vi "Format Main Status.vi"() -> (2 "FullStat":string, 3 "ShortStat":string)   [LabVIEW 2019]
uses:
  RT Controls/Top Dome Status.ctl
  RT Controls/Main Box Status.ctl
  RT Controls/Rotation Status.ctl
  RT Controls/Last Rotation.ctl
  RT Controls/Homing State.ctl
  RT Controls/Main Box Control.ctl
  RT Controls/Top Dome Control.ctl
  RT Controls/Main Box Config.ctl
  RT Controls/TopBox Config.ctl
  RT Controls/FPGA State.ctl
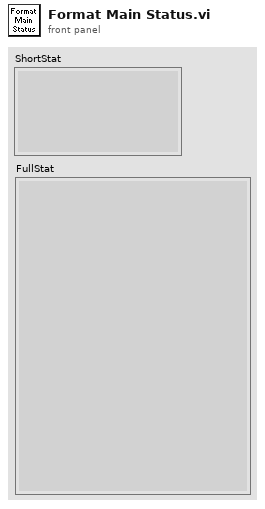
[diagram p1: front panel]
types:
  T1 = typedef "Main Box Config.ctl" = cluster{"WatchdogTim":i32, "DirRevDel":i32, "Coast":dbl, "HSThres":dbl, "EncCounts360":u64, "HomePos":dbl, "EncRefDeg":dbl, "EncRefCounts":u64, "Tol":dbl, "CloudEn":bool, "AutoShutEn":bool, "RainTim":i32, "AZTimeout":i32, "AZEncPol":enum16{"Positive", "Negative"}}
  T2 = typedef "Main Box Status.ctl" = cluster{"RotStatus":T3, "EMButton":bool, "TopComms":bool, "CurAZ":dbl, "At Home":bool, "LastRot":T4, "Cloud":bool, "CurAZEnc":u64, "LastAZ":dbl, "AutoShut":bool, "WDTime":bool, "HomeState":T5}
  T3 = typedef "Rotation Status.ctl" = enum16{"Stop", "Left", "Right", "Homing"}
  T4 = typedef "Last Rotation.ctl" = enum16{"--", "RR", "RL"}
  T5 = typedef "Homing State.ctl" = enum16{"Idle", "SlewFwd", "SlewRev", "SeekFwd", "SeekRev", "AtHome", "FwdWait", "RevWait"}
  T6 = typedef "Top Dome Status.ctl" = cluster{"UpperDoorStatus":enum16{"Ajar", "Open", "Shut", "Error"}, "LowerDoorStatus":enum16{"Ajar", "Shut", "Open", "Error"}, "EM Button":bool, "WDTime":bool, "AutoShut":bool, "Rain":bool, "Interlock":bool, "UpperDoorEl":dbl, "LowerDoorEl":dbl, "UpperDoorEnc":u64, "LowerDoorEnc":u64}
  T7 = typedef "Top Dome Control.ctl" = cluster{"OpenLowerDoor":bool, "CloseLowerDoor":bool, "OpenMainDoor":bool, "CloseMainDoor":bool}
  T8 = typedef "Main Box Control.ctl" = cluster{"ForwardDome":bool, "ReverseDome":bool, "GotoHome":bool, "HighSpeed":bool}
  T9 = typedef "FPGA State.ctl" = cluster{"mode request":enum16{"stop", "home", "position", "center"}, "az last rotation":enum16{"none", "forward", "reverse"}, "emergency stop":bool, "error?":bool, "errors":cluster{"emergency stop":bool, "encoder":bool, "az timeout":bool, "m1":bool, "m2":bool, "m4":bool}, "az enc counts":u64, "az pos":fxp<+/-,32,2>, "mode":u8, "sub mode":u8, "enc status":u16, "buttons":cluster{"em-stop":bool, "forward":bool, "reverse":bool, "open":bool, "close":bool, "up":bool, "down":bool, "force stop":bool}, "cloud?":bool, "cloud to counter":u32, "az to counter":u32, "env sensor":bool, "home sensor":bool, "rev dly counter":u32, "cmd request":i8, "cmd":i8, "config":cluster{"io.cloud-enable":bool, "io.encoder-negate":bool, "io.encoder-ref":u64, "io.encoder-step":u64, "io.home-pos":fxp<+/-,32,2>, "sm.az-timeout (ms)":u32, "sm.encoder-no-error":u16, "sm.main-pos-hs-thres":fxp<+/-,32,2>, "sm.main-pos-tol":fxp<+/-,32,2>, "sm.cloud-timeout (ms)":u32, "sm.rev-dly (ms)":u32, "io.encoder-center":u64, "sm-main-center-hs-thres":u64, "sm-main-center-tol":u64}, "homing?":bool, "homed?":bool, "az pos req":fxp<+/-,32,2>, "homing wait counter":u32, "config out":cluster{"io.cloud-enable":bool, "io.encoder-negate":bool, "io.encoder-ref":u64, "io.encoder-step":u64, "io.home-pos":fxp<+/-,32,2>, "sm.az-timeout (ms)":u32, "sm.encoder-no-error":u16, "sm.main-pos-hs-thres":fxp<+/-,32,2>, "sm.main-pos-tol":fxp<+/-,32,2>, "sm.cloud-timeout (ms)":u32, "sm.rev-dly (ms)":u32, "io.encoder-center":u64, "sm-main-center-hs-thres":u64, "sm-main-center-tol":u64}, "Chassis Temperature":i16}
  T10 = typedef "TopBox Config.ctl" = cluster{"WatchdogTim":i32, "RainEn":bool, "DoorMoveTO":i32, "AutoShutEn":bool, "DirRevDel":i32, "UpperClosedEnc":u64, "UpperOpenEnc":u64, "LowerClosedEnc":u64, "LowerOpenEnc":u64, "RainTim":i32, "DropoutTim":i32}
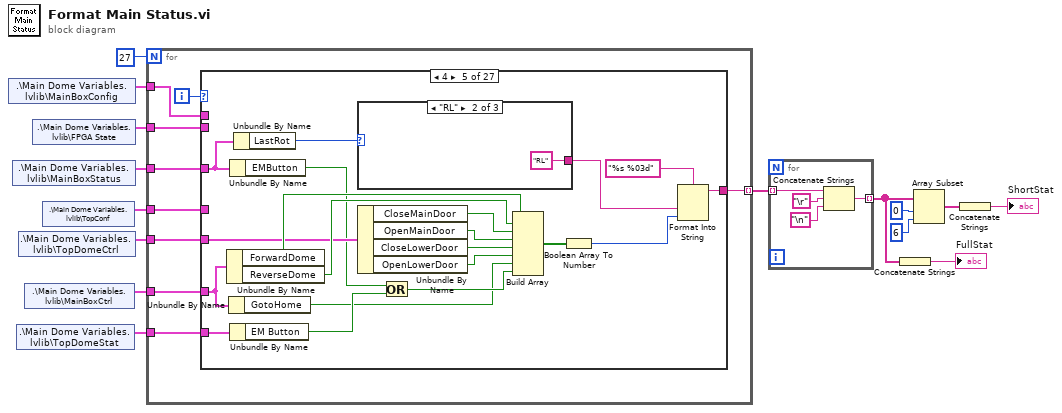
[diagram p0: block diagram]
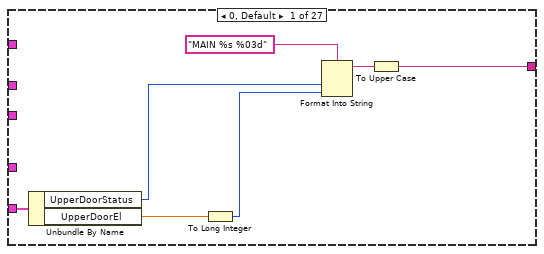
[diagram p2: hidden frame]
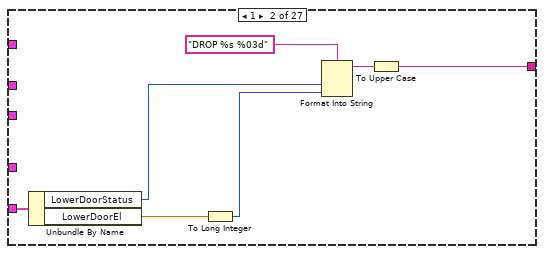
[diagram p3: hidden frame]
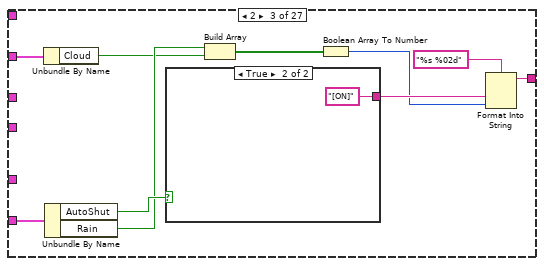
[diagram p4: hidden frame]
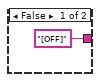
[diagram p5: hidden frame]
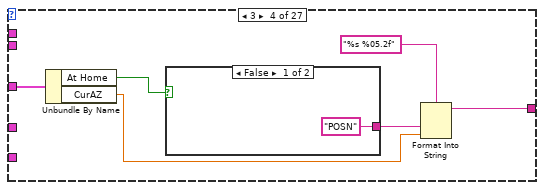
[diagram p6: hidden frame]
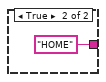
[diagram p7: hidden frame]
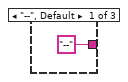
[diagram p8: hidden frame]
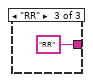
[diagram p9: hidden frame]
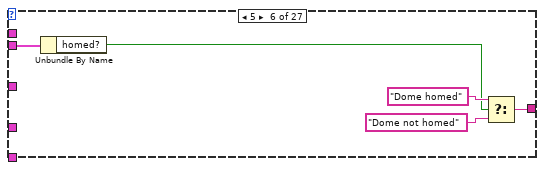
[diagram p10: hidden frame]
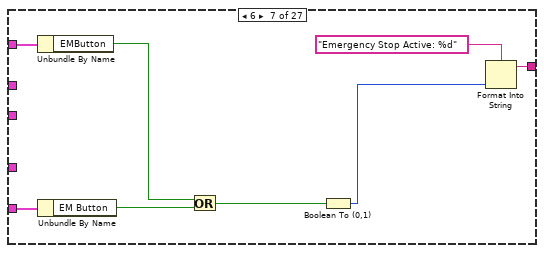
[diagram p11: hidden frame]
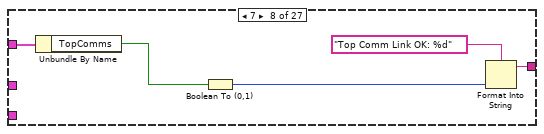
[diagram p12: hidden frame]
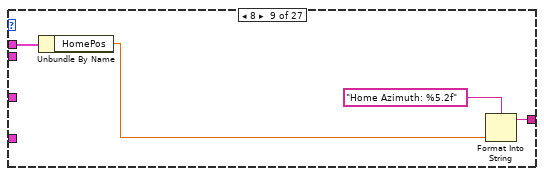
[diagram p13: hidden frame]
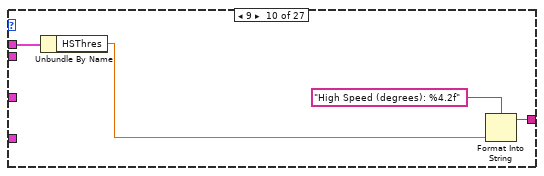
[diagram p14: hidden frame]
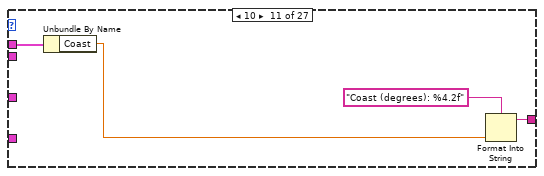
[diagram p15: hidden frame]
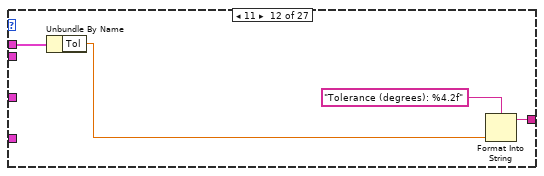
[diagram p16: hidden frame]
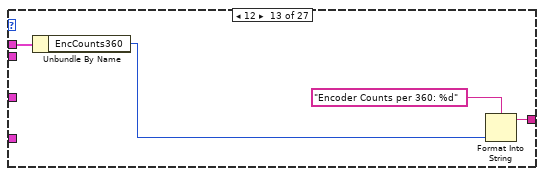
[diagram p17: hidden frame]
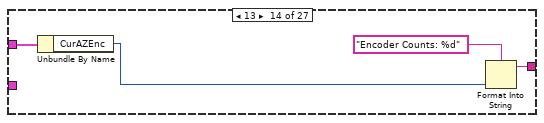
[diagram p18: hidden frame]
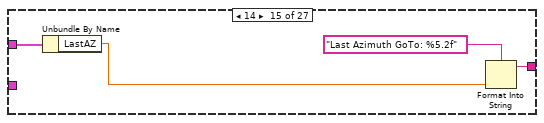
[diagram p19: hidden frame]
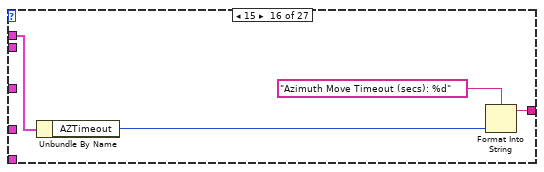
[diagram p20: hidden frame]
diagram:
  n1 = shared-variable ".\\Main Dome Variables.lvlib\\MainBoxConfig"() -> (w11:T1)  [unwired: 1 in, 1 out]
  n2 = shared-variable ".\\Main Dome Variables.lvlib\\MainBoxStatus"() -> (w14:T2)  [unwired: 1 in, 1 out]
  n3 = shared-variable ".\\Main Dome Variables.lvlib\\TopDomeStat"() -> (w15:T6)  [unwired: 1 in, 1 out]
  n4 = shared-variable ".\\Main Dome Variables.lvlib\\TopDomeCtrl"() -> (w12:T7)  [unwired: 1 in, 1 out]
  n5 = shared-variable ".\\Main Dome Variables.lvlib\\MainBoxCtrl"() -> (w13:T8)  [unwired: 1 in, 1 out]
  n6 = shared-variable ".\\Main Dome Variables.lvlib\\FPGA State"() -> (w1:T9)  [unwired: 1 in, 1 out]
  n7 = shared-variable ".\\Main Dome Variables.lvlib\\TopConf"() -> (w10:T10)  [unwired: 1 in, 1 out]
  n8 = for {
    N: 27 -> [_]
    tunnel: w15 -> [w24]
    tunnel: [w22] -> w5 mode=indexing
    tunnel: w14 -> [w21]
    tunnel: w13 -> [w20]
    tunnel: w12 -> [w19]
    tunnel: w11 -> [w18]
    tunnel: w10 -> [w17]
    tunnel: w1 -> [w16]
    i -> [w23]
    n9 = case shown="4" w23 {
      tunnel: w24 -> [w31 w38 w48 _ w67 _ w91 _ _ _ _ _ _ _ _ _ w134 _ _ _ _ _ _ _ _ _ _]
      tunnel: [w28 w35 w43 w51 w64 w85 w93 w98 w102 w106 w110 w114 w118 w122 w126 w130 w135 w140 w144 w148 w152 w156 w160 w164 w168 w172 w175] -> w22
      tunnel: w21 -> [_ _ w45 w56 w62 _ w92 w97 _ _ _ _ _ w120 w124 _ _ _ _ _ _ _ _ _ _ _ _]
      tunnel: w20 -> [_ _ _ _ w60 _ _ _ _ _ _ _ _ _ _ _ _ _ _ _ _ _ _ _ _ _ _]
      tunnel: w19 -> [_ _ _ _ w69 _ _ _ _ _ _ _ _ _ _ _ _ _ _ _ _ _ _ _ _ _ _]
      tunnel: w18 -> [_ _ _ _ _ _ _ _ w101 w105 w109 w113 w117 _ _ w128 _ w137 _ _ _ _ _ _ _ _ _]
      tunnel: w17 -> [_ _ _ _ _ _ _ _ _ _ _ _ _ _ _ _ _ _ w143 w147 w151 w155 w159 w163 w167 w171 _]
      tunnel: w16 -> [_ _ _ _ _ w83 _ _ _ _ _ _ _ _ _ _ _ _ _ _ _ _ _ _ _ _ w174]
      frame 0, Default {
        n10 = Unbundle By Name(w31) -> ("UpperDoorStatus"=w27:enum16{"Ajar", "Open", "Shut", "Error"}, "UpperDoorEl"=w26:dbl)
        n11 = To Long Integer(number=w26) -> (32bit integer=w25:i32)
        n12 = Format Into String(format string="MAIN %s %03d", w27, w25) -> (resulting string=w29:string)  [unwired: 2 in, 1 out]
        n13 = To Upper Case(1:w29) -> (0:w28:string)
      }
      frame 1 {
        n14 = Unbundle By Name(w38) -> ("LowerDoorStatus"=w34:enum16{"Ajar", "Shut", "Open", "Error"}, "LowerDoorEl"=w33:dbl)
        n15 = To Long Integer(number=w33) -> (32bit integer=w32:i32)
        n16 = Format Into String(format string="DROP %s %03d", w34, w32) -> (resulting string=w36:string)  [unwired: 2 in, 1 out]
        n17 = To Upper Case(1:w36) -> (0:w35:string)
      }
      frame 2 {
        n18 = Unbundle By Name(w45) -> ("Cloud"=w40:bool)
        n19 = Unbundle By Name(w48) -> ("AutoShut"=w47:bool, "Rain"=w41:bool)
        n20 = case shown="True" w47 {
          tunnel: ["[OFF]" ("string") "[ON]" ("string")] -> w44
          frame False {
          }
          frame True {
          }
        }
        n21 = Build Array(w41, w40) -> (w42:bool[])
        n22 = Boolean Array To Number(Boolean array=w42) -> (number=w39:u32)
        n23 = Format Into String(format string="%s %02d", w44, w39) -> (resulting string=w43:string)  [unwired: 2 in, 1 out]
      }
      frame 3 {
        n24 = Unbundle By Name(w56) -> ("At Home"=w55:bool, "CurAZ"=w52:dbl)
        n25 = case shown="False" w55 {
          tunnel: ["POSN" ("string") "HOME" ("string")] -> w54
          frame False {
          }
          frame True {
          }
        }
        n26 = Format Into String(format string="%s %05.2f", w54, w52) -> (resulting string=w51:string)  [unwired: 2 in, 1 out]
      }
      frame 4 {
        n27 = Unbundle By Name(w60) -> ("ForwardDome"=w75:bool, "ReverseDome"=w74:bool)
        n28 = Unbundle By Name(w60) -> ("GotoHome"=w59:bool)
        n29 = Unbundle By Name(w62) -> ("EMButton"=w61:bool)
        n30 = Unbundle By Name(w67) -> ("EM Button"=w63:bool)
        n31 = Unbundle By Name(w62) -> ("LastRot"=w78:T4)
        n32 = case shown="\"RL\"" w78 {
          tunnel: ["--" ("string") "RL" ("string") "RR" ("string")] -> w76
          frame "--", Default {
          }
          frame "RL" {
          }
          frame "RR" {
          }
        }
        n33 = Unbundle By Name(w69) -> ("CloseMainDoor"=w73:bool, "OpenMainDoor"=w72:bool, "CloseLowerDoor"=w71:bool, "OpenLowerDoor"=w70:bool)
        n34 = Or(x=w61, y=w63) -> (x .or. y?=w68:bool)
        n35 = Build Array(w75, w74, w73, w72, w71, w70, w59, w68) -> (w66:bool[])
        n36 = Boolean Array To Number(Boolean array=w66) -> (number=w65:u32)
        n37 = Format Into String(format string="%s %03d", w76, w65) -> (resulting string=w64:string)  [unwired: 2 in, 1 out]
      }
      frame 5 {
        n38 = Unbundle By Name(w83) -> ("homed?"=w82:bool)
        n39 = Select(t="Dome homed", s=w82, f="Dome not homed") -> (s? t:f=w85:string)
      }
      frame 6 {
        n40 = Unbundle By Name(w92) -> ("EMButton"=w88:bool)
        n41 = Unbundle By Name(w91) -> ("EM Button"=w87:bool)
        n42 = Or(x=w88, y=w87) -> (x .or. y?=w90:bool)
        n43 = Boolean To (0,1)(Boolean=w90) -> (0, 1=w89:i16)
        n44 = Format Into String(format string="Emergency Stop Active: %d", w89) -> (resulting string=w93:string)  [unwired: 2 in, 1 out]
      }
      frame 7 {
        n45 = Unbundle By Name(w97) -> ("TopComms"=w95:bool)
        n46 = Boolean To (0,1)(Boolean=w95) -> (0, 1=w96:i16)
        n47 = Format Into String(format string="Top Comm Link OK: %d", w96) -> (resulting string=w98:string)  [unwired: 2 in, 1 out]
      }
      frame 8 {
        n48 = Unbundle By Name(w101) -> ("HomePos"=w100:dbl)
        n49 = Format Into String(format string="Home Azimuth: %5.2f", w100) -> (resulting string=w102:string)  [unwired: 2 in, 1 out]
      }
      frame 9 {
        n50 = Unbundle By Name(w105) -> ("HSThres"=w104:dbl)
        n51 = Format Into String(format string="High Speed (degrees): %4.2f", w104) -> (resulting string=w106:string)  [unwired: 2 in, 1 out]
      }
      frame 10 {
        n52 = Unbundle By Name(w109) -> ("Coast"=w108:dbl)
        n53 = Format Into String(format string="Coast (degrees): %4.2f", w108) -> (resulting string=w110:string)  [unwired: 2 in, 1 out]
      }
      frame 11 {
        n54 = Unbundle By Name(w113) -> ("Tol"=w112:dbl)
        n55 = Format Into String(format string="Tolerance (degrees): %4.2f", w112) -> (resulting string=w114:string)  [unwired: 2 in, 1 out]
      }
      frame 12 {
        n56 = Unbundle By Name(w117) -> ("EncCounts360"=w116:u64)
        n57 = Format Into String(format string="Encoder Counts per 360: %d", w116) -> (resulting string=w118:string)  [unwired: 2 in, 1 out]
      }
      frame 13 {
        n58 = Unbundle By Name(w120) -> ("CurAZEnc"=w121:u64)
        n59 = Format Into String(format string="Encoder Counts: %d", w121) -> (resulting string=w122:string)  [unwired: 2 in, 1 out]
      }
      frame 14 {
        n60 = Unbundle By Name(w124) -> ("LastAZ"=w125:dbl)
        n61 = Format Into String(format string="Last Azimuth GoTo: %5.2f", w125) -> (resulting string=w126:string)  [unwired: 2 in, 1 out]
      }
      frame 15 {
        n62 = Unbundle By Name(w128) -> ("AZTimeout"=w129:i32)
        n63 = Format Into String(format string="Azimuth Move Timeout (secs): %d", w129) -> (resulting string=w130:string)  [unwired: 2 in, 1 out]
      }
      frame 16 {
        n64 = Unbundle By Name(w134) -> ("Rain"=w133:bool)
        n65 = Boolean To (0,1)(Boolean=w133) -> (0, 1=w132:i16)
        n66 = Format Into String(format string="Rain-Snow enabled: %d", w132) -> (resulting string=w135:string)  [unwired: 2 in, 1 out]
      }
      frame 17 {
        n67 = Unbundle By Name(w137) -> ("CloudEn"=w139:bool)
        n68 = Boolean To (0,1)(Boolean=w139) -> (0, 1=w138:i16)
        n69 = Format Into String(format string="Cloud Sensor enabled: %d", w138) -> (resulting string=w140:string)  [unwired: 2 in, 1 out]
      }
      frame 18 {
        n70 = Unbundle By Name(w143) -> ("WatchdogTim"=w142:i32)
        n71 = Format Into String(format string="Watchdog Reset Time: %d", w142) -> (resulting string=w144:string)  [unwired: 2 in, 1 out]
      }
      frame 19 {
        n72 = Unbundle By Name(w147) -> ("DropoutTim"=w146:i32)
        n73 = Format Into String(format string="Dropout Timer: %d", w146) -> (resulting string=w148:string)  [unwired: 2 in, 1 out]
      }
      frame 20 {
        n74 = Unbundle By Name(w151) -> ("DirRevDel"=w150:i32)
        n75 = Format Into String(format string="Reverse Delay: %d", w150) -> (resulting string=w152:string)  [unwired: 2 in, 1 out]
      }
      frame 21 {
        n76 = Unbundle By Name(w155) -> ("UpperClosedEnc"=w154:u64)
        n77 = Format Into String(format string="Main Door Encoder Closed: %d", w154) -> (resulting string=w156:string)  [unwired: 2 in, 1 out]
      }
      frame 22 {
        n78 = Unbundle By Name(w159) -> ("UpperOpenEnc"=w158:u64)
        n79 = Format Into String(format string="Main Door Encoder Opened: %d", w158) -> (resulting string=w160:string)  [unwired: 2 in, 1 out]
      }
      frame 23 {
        n80 = Unbundle By Name(w163) -> ("LowerClosedEnc"=w162:u64)
        n81 = Format Into String(format string="Dropout Encoder Closed: %d", w162) -> (resulting string=w164:string)  [unwired: 2 in, 1 out]
      }
      frame 24 {
        n82 = Unbundle By Name(w167) -> ("LowerOpenEnc"=w166:u64)
        n83 = Format Into String(format string="Dropout Encoder Opened: %d", w166) -> (resulting string=w168:string)  [unwired: 2 in, 1 out]
      }
      frame 25 {
        n84 = Unbundle By Name(w171) -> ("DoorMoveTO"=w170:i32)
        n85 = Format Into String(format string="Door Move Timeout (secs): %d", w170) -> (resulting string=w172:string)  [unwired: 2 in, 1 out]
      }
      frame 26 {
        n86 = Unbundle By Name(w174) -> ("homed?"=w180:bool)
        n87 = Select(t="True", s=w180, f="False") -> (s? t:f=w176:string)
        n88 = Format Into String(format string="Dome has been homed: %s", w176) -> (resulting string=w175:string)  [unwired: 2 in, 1 out]
      }
    }
  }
  n89 = for {
    tunnel: w5 -> [w184] mode=indexing
    tunnel: [w181] -> w3 mode=indexing
    n90 = Concatenate Strings(w184, "\r", "\n") -> (w181:string)
  }
  n91 = Concatenate Strings(w3) -> (→"FullStat":string)
  n92 = Array Subset(array=w3, index=0, length=6) -> (w2:string[])
  n93 = Concatenate Strings(w2) -> (→"ShortStat":string)
